vi "Delta_P_set_neg_to_zero.vi"() -> (5 "Plug in titles":string[](array[string]), 7 "Plug in values":string[](array[string]))   [LabVIEW 2010]
uses:
  Globals/Plug_in_data_global.vi
  Globals/Meas_global.vi
panel:
  out "D,D/2":dbl[](graph)
  out "Flange":dbl[](graph)
  out "Corner":dbl[](graph)
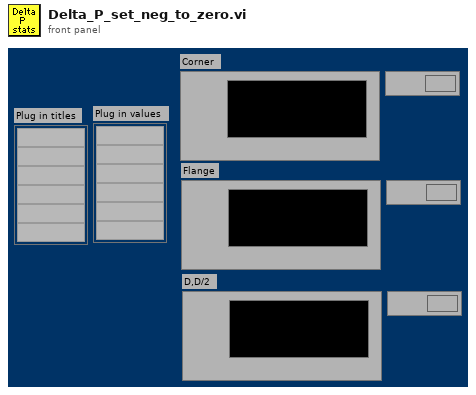
[diagram p1: front panel]
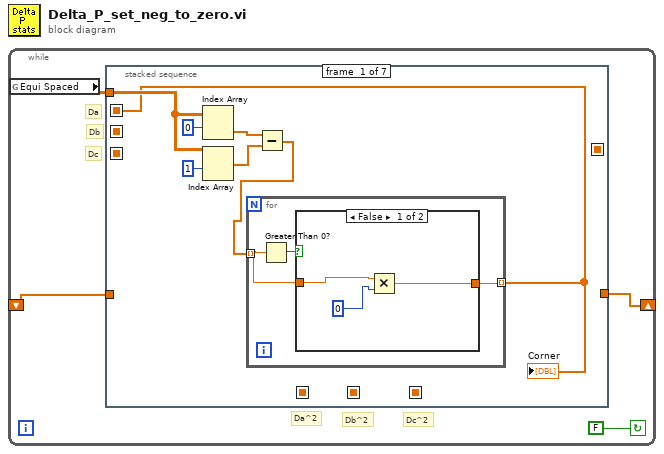
[diagram p0: block diagram]
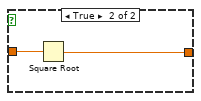
[diagram p2: hidden frame]
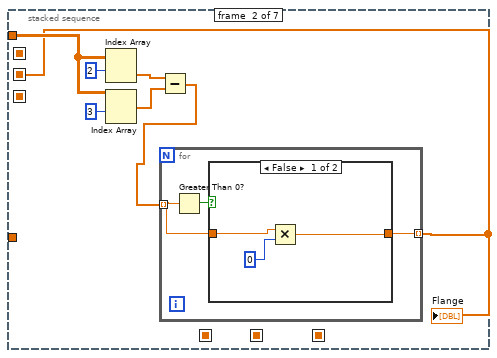
[diagram p3: hidden frame]
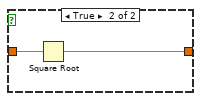
[diagram p4: hidden frame]
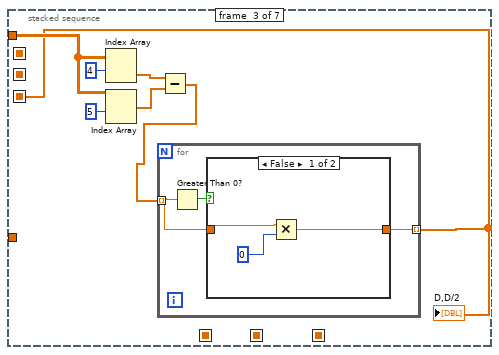
[diagram p5: hidden frame]
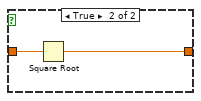
[diagram p6: hidden frame]
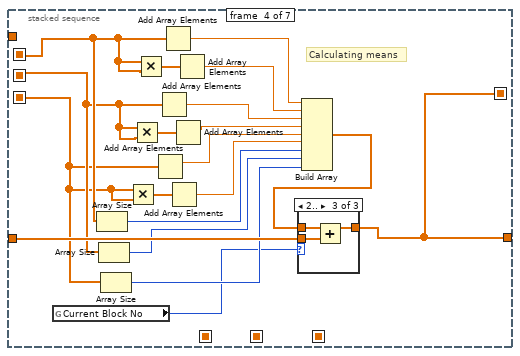
[diagram p7: hidden frame]
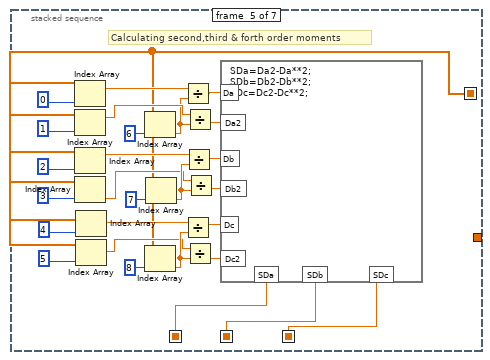
[diagram p10: hidden frame]
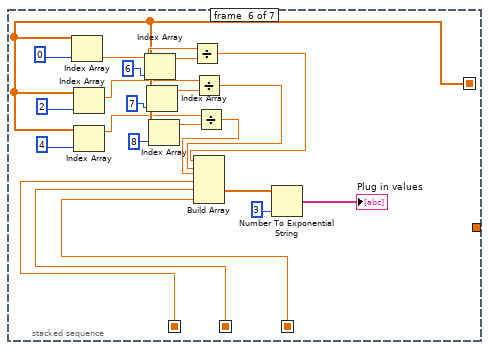
[diagram p11: hidden frame]
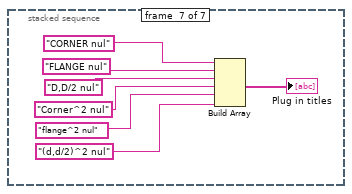
[diagram p12: hidden frame]
diagram:
  n1 = while {
    shift-left: _ -> [w4]
    shift-right: [w3] -> _
    stop <- FALSE continue-if-true
    # "Dc^2"
    # "Db^2"
    # "Da^2"
    # "Dc"
    # "Db"
    # "Da"
    n2 = global read "Plug_in_data_global.vi" "Equi Spaced"() -> (w2:dbl[][])
    n3 = stacked-sequence {
      seq-local: [_ _ _ _ w94 _ _] -> [_ _ _ _ _ w122 _]
      seq-local: [_ _ _ w52 _ _ _] -> [_ _ _ _ w78 w106 _]
      seq-local: [_ _ _ _ w95 _ _] -> [_ _ _ _ _ w123 _]
      seq-local: [_ _ _ _ w93 _ _] -> [_ _ _ _ _ w119 _]
      seq-local: [w5 _ _ _ _ _ _] -> [_ _ _ w57 _ _ _]
      seq-local: [_ w20 _ _ _ _ _] -> [_ _ _ w56 _ _ _]
      seq-local: [_ _ w35 _ _ _ _] -> [_ _ _ w55 _ _ _]
      tunnel: w4 -> [_ _ _ w66 _ _ _]
      tunnel: [_ _ _ w52 _ _ _] -> w3
      tunnel: w2 -> [w7 w22 w37 _ _ _ _]
      frame #0 {
        n4 = Index Array(array=w7, index (row)=0) -> (element=w9:dbl[])  [unwired: 1 in]
        n5 = Index Array(array=w7, index (row)=1) -> (element=w8:dbl[])  [unwired: 1 in]
        n6 = Subtract(x=w9, y=w8) -> (x-y=w6:dbl[])
        n7 = for {
          tunnel: w6 -> [w13] mode=indexing
          tunnel: [w12] -> w5 mode=indexing
          n8 = Greater Than 0?(x=w13) -> (x > 0?=w14:bool)
          n9 = case shown="False" w14 {
            tunnel: w13 -> [w17 w19]
            tunnel: [w15 w18] -> w12
            frame False {
              n10 = Multiply(x=w17, y=0) -> (x*y=w15:dbl)
            }
            frame True {
              n11 = Square Root(x=w19) -> (sqrt(x)=w18:dbl)
            }
          }
        }
        "Corner" <- w5
      }
      frame #1 {
        n12 = Index Array(array=w22, index (row)=2) -> (element=w24:dbl[])  [unwired: 1 in]
        n13 = Index Array(array=w22, index (row)=3) -> (element=w23:dbl[])  [unwired: 1 in]
        n14 = Subtract(x=w24, y=w23) -> (x-y=w21:dbl[])
        n15 = for {
          tunnel: w21 -> [w28] mode=indexing
          tunnel: [w27] -> w20 mode=indexing
          n16 = Greater Than 0?(x=w28) -> (x > 0?=w29:bool)
          n17 = case shown="False" w29 {
            tunnel: w28 -> [w32 w34]
            tunnel: [w30 w33] -> w27
            frame False {
              n18 = Multiply(x=w32, y=0) -> (x*y=w30:dbl)
            }
            frame True {
              n19 = Square Root(x=w34) -> (sqrt(x)=w33:dbl)
            }
          }
        }
        "Flange" <- w20
      }
      frame #2 {
        n20 = Index Array(array=w37, index (row)=4) -> (element=w39:dbl[])  [unwired: 1 in]
        n21 = Index Array(array=w37, index (row)=5) -> (element=w38:dbl[])  [unwired: 1 in]
        n22 = Subtract(x=w39, y=w38) -> (x-y=w36:dbl[])
        n23 = for {
          tunnel: w36 -> [w43] mode=indexing
          tunnel: [w42] -> w35 mode=indexing
          n24 = Greater Than 0?(x=w43) -> (x > 0?=w44:bool)
          n25 = case shown="False" w44 {
            tunnel: w43 -> [w47 w49]
            tunnel: [w45 w48] -> w42
            frame False {
              n26 = Multiply(x=w47, y=0) -> (x*y=w45:dbl)
            }
            frame True {
              n27 = Square Root(x=w49) -> (sqrt(x)=w48:dbl)
            }
          }
        }
        "D,D/2" <- w35
      }
      frame #3 {
        # "Calculating means"
        n28 = global read "Meas_global.vi" "Current Block No"() -> (w51:i32)
        n29 = Array Size(array=w57) -> (size(s)=w58:i32)
        n30 = Array Size(array=w56) -> (size(s)=w54:i32)
        n31 = Array Size(array=w55) -> (size(s)=w53:i32)
        n32 = Multiply(x=w55, y=w55) -> (x*y=w63:dbl[])
        n33 = Multiply(x=w56, y=w56) -> (x*y=w64:dbl[])
        n34 = Multiply(x=w57, y=w57) -> (x*y=w65:dbl[])
        n35 = Add Array Elements(numeric array=w55) -> (sum=w60:dbl)
        n36 = Add Array Elements(numeric array=w56) -> (sum=w62:dbl)
        n37 = Add Array Elements(numeric array=w57) -> (sum=w68:dbl)
        n38 = Add Array Elements(numeric array=w63) -> (sum=w59:dbl)
        n39 = Add Array Elements(numeric array=w64) -> (sum=w61:dbl)
        n40 = Add Array Elements(numeric array=w65) -> (sum=w67:dbl)
        n41 = Build Array(w68, w67, w62, w61, w60, w59, w58, w54, w53) -> (w50:dbl[])
        n42 = case shown="2.." w51 {
          tunnel: [w69 w70 w73] -> w52
          tunnel: w66 -> [_ _ w72]
          tunnel: w50 -> [w69 w70 w71]
          frame ..0 {
          }
          frame 1 {
          }
          frame 2.. {
            n43 = Add(x=w71, y=w72) -> (x+y=w73:dbl[])
          }
        }
      }
      frame #4 {
        # "Calculating second,third & forth order moments"
        n44 = Index Array(array=w78, index=0) -> (element=w90:dbl)
        n45 = Index Array(array=w78, index=1) -> (element=w91:dbl)
        n46 = Index Array(array=w78, index=2) -> (element=w82:dbl)
        n47 = Index Array(array=w78, index=3) -> (element=w81:dbl)
        n48 = Index Array(array=w78, index=4) -> (element=w80:dbl)
        n49 = Index Array(array=w78, index=5) -> (element=w79:dbl)
        n50 = Index Array(array=w78, index=6) -> (element=w89:dbl)
        n51 = Index Array(array=w78, index=8) -> (element=w83:dbl)
        n52 = Index Array(array=w78, index=7) -> (element=w86:dbl)
        n53 = Divide(x=w90, y=w89) -> (x/y=w88:dbl)
        n54 = Divide(x=w80, y=w83) -> (x/y=w76:dbl)
        n55 = Divide(x=w82, y=w86) -> (x/y=w74:dbl)
        n56 = Divide(x=w91, y=w89) -> (x/y=w87:dbl)
        n57 = Divide(x=w79, y=w83) -> (x/y=w77:dbl)
        n58 = Divide(x=w81, y=w86) -> (x/y=w75:dbl)
        n59 = formula code="SDa=Da2-Da**2;\nSDb=Db2-Db**2;\nSDc=Dc2-Dc**2;"("Da2"=w87, "Da"=w88, "Db"=w74, "Db2"=w75, "Dc"=w76, "Dc2"=w77) -> ("SDa"=w95:dbl, "SDb"=w94:dbl, "SDc"=w93:dbl)
      }
      frame #5 {
        n60 = Index Array(array=w106, index=0) -> (element=w112:dbl)
        n61 = Index Array(array=w106, index=2) -> (element=w104:dbl)
        n62 = Index Array(array=w106, index=4) -> (element=w105:dbl)
        n63 = Index Array(array=w106, index=6) -> (element=w113:dbl)
        n64 = Index Array(array=w106, index=7) -> (element=w110:dbl)
        n65 = Index Array(array=w106, index=8) -> (element=w107:dbl)
        n66 = Divide(x=w112, y=w113) -> (x/y=w111:dbl)
        n67 = Divide(x=w104, y=w110) -> (x/y=w103:dbl)
        n68 = Divide(x=w105, y=w107) -> (x/y=w102:dbl)
        n69 = Build Array(w111, w103, w102, w123, w122, w119) -> (w120:dbl[])
        n70 = Number To Exponential String(number=w120, precision (6)=3) -> (E-format string=→"Plug in values":string[])  [unwired: 2 in]
      }
      frame #6 {
        n71 = Build Array("CORNER nul", "FLANGE nul", "D,D/2 nul", "Corner^2 nul", "flange^2 nul", "(d,d/2)^2 nul") -> (→"Plug in titles":string[])
      }
    }
  }
